vi "vlc_load_test.vi"() -> ()   [LabVIEW 2018]
panel:
  out "Status":string="5: Wait"
  in  "delay (ms)":u32=100
  in  "Abort":bool
  out "Iteration":i32=154
  in  "Operation":T1(ring)
  in  "video_capture_dir":path=path "D:/ReLOAD_Working/video_testing"
  in  "VLC command":string="dshow:// :dshow-vdev~\"\" :dshow-adev~\"none\" :dshow-size~\"320x240\" :dshow-caching~80 :dshow-fps~30.000000 --sub-filter logo:time --logo-file \"LOGO_FILE\" --logo-position~9 --time-position~10 -I http :sout~#transcode{vcodec~FLV1,vb~256,scale~1,venc~ffmpeg{keyint~30},acodec~none,sfilter~logo:time}:std{access~file,mux~ffmpeg{mux~flv},dst~\"FILENAME.flv\"}"
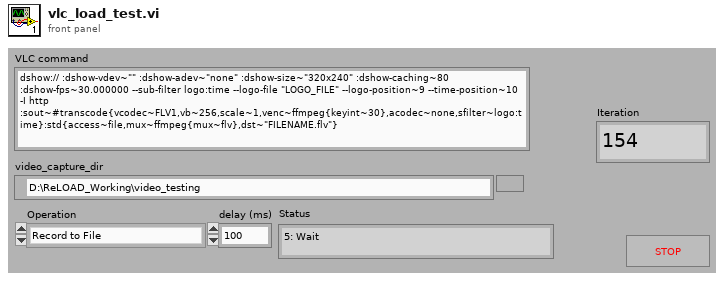
[diagram p1: front panel]
types:
  T1 = enum16{"Record to File", "Preview 320x240", "Preview 640x480"}
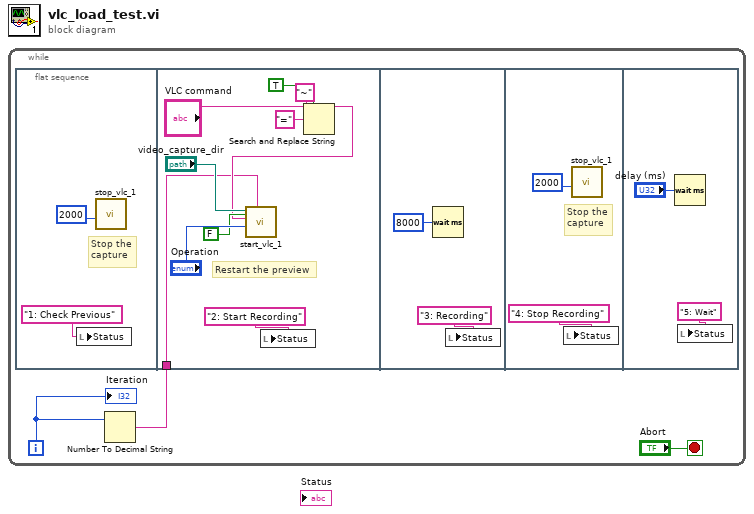
[diagram p0: block diagram]
diagram:
  n1 = while {
    i -> [w3]
    stop <- "Abort" stop-if-true
    n2 = flat-sequence {
      tunnel: w2 -> [w7]
      frame #0 {
        # "Stop the\ncapture"
        n3 = local write "Status"("1: Check Previous" ("Status")) -> ()
        n4 = call "stop_vlc_1.vi"("Timeout (ms)"=2000) -> ()  [unwired: 10 in, 1 out]
      }
      frame #1 {
        # "Restart the preview"
        n5 = local write "Status"("2: Start Recording" ("Status")) -> ()
        n6 = Search and Replace String(replace all?=TRUE ("replace all? (F)"), input string="VLC command", search string="~", replace string="=" ("replace string (\"\")")) -> (result string=w8:string)  [unwired: 1 in, 6 out]
        n7 = call "start_vlc_1.vi"("Timestamp"=w7, "wait until completion? (T)"=FALSE, "Operation"="Operation", "VLC command"=w8, "video_capture_dir"="video_capture_dir") -> ()  [unwired: 4 in, 3 out]
      }
      frame #2 {
        n8 = Wait (ms)(milliseconds to wait=u32 8000) -> ()  [unwired: 1 out]
        n9 = local write "Status"("3: Recording" ("Status")) -> ()
      }
      frame #3 {
        # "Stop the\ncapture"
        n10 = local write "Status"("4: Stop Recording" ("Status")) -> ()
        n11 = call "stop_vlc_1.vi"("Timeout (ms)"=2000) -> ()  [unwired: 10 in, 1 out]
      }
      frame #4 {
        n12 = Wait (ms)(milliseconds to wait="delay (ms)") -> ()  [unwired: 1 out]
        n13 = local write "Status"("5: Wait" ("Status")) -> ()
      }
    }
    n14 = Number To Decimal String(number=w3) -> (decimal integer string=w2:string)  [unwired: 1 out]
    "Iteration" <- w3
  }
